vi "FTW-Project-ConditionalDisableSymbols-Set.vi"(0 "Project Ref (blank for Active Project)":refnum<vi>, 5 "Target (Root or My Computer)":string(combo)="Root", 7 "Conditional Disable Symbol":string, 9 "Value":string, 11 "error in":errorcluster) -> (4 "Project out":refnum<vi>, 6 "Conditional Disable Symbols out":variant, 15 "error out":errorcluster)   [LabVIEW 2012]
doc: "This VI will add to or modify existing Conditional Disable Symbols. It will not remove existing Conditional Disable Symbols."
panel:
  # "Inputs"
  # "Outputs"
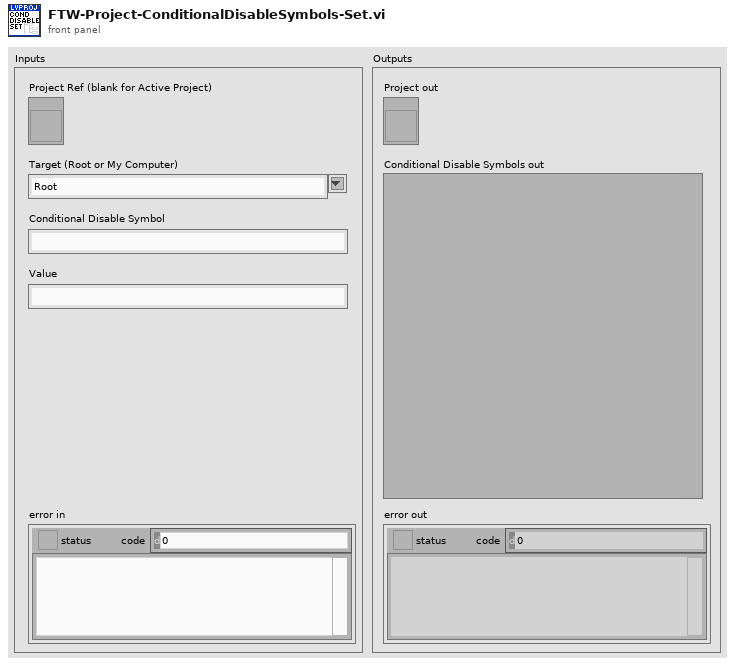
[diagram p1: front panel]
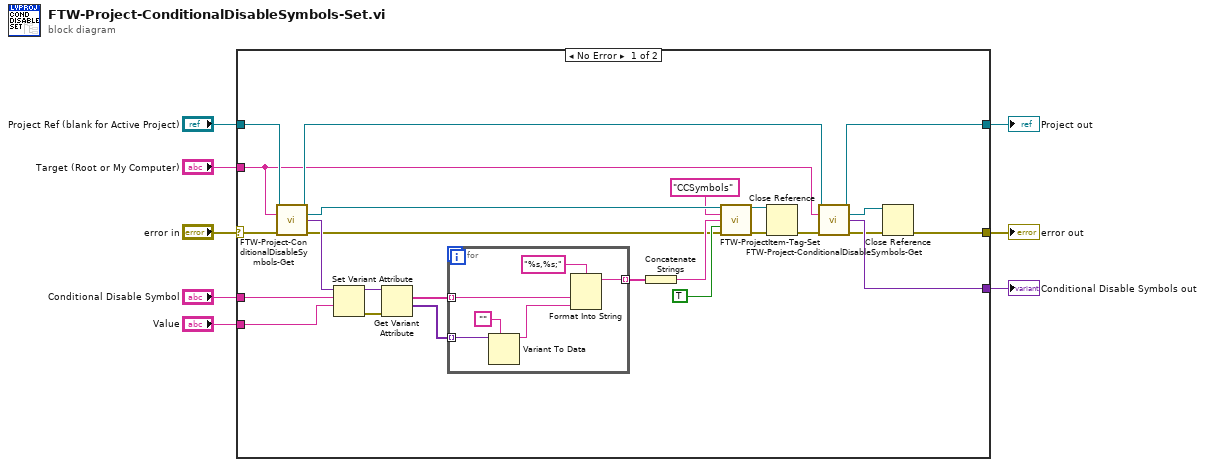
[diagram p0: block diagram]
diagram:
  n1 = case shown="No Error" "error in" {
    selector: "error in" -> [w32 w41]
    tunnel: [w19 w41] -> w8
    tunnel: "Target (Root or My Computer)" -> [w23 _]
    tunnel: "Project Ref (blank for Active Project)" -> [w33 w40]
    tunnel: [w25 w40] -> w4
    tunnel: [w22 _] -> w3
    tunnel: "Conditional Disable Symbol" -> [w18 _]
    tunnel: "Value" -> [w17 _]
    frame No Error {
      n2 = call "FTW-Project-ConditionalDisableSymbols-Get.vi"("Project Ref (blank for Active Project)"=w33, "Target (Root or My Computer)"=w23, "error in"=w32) -> ("Project out"=w26:refnum<vi>, "TargetItem out"=w16:refnum<vi>, "Conditional Disable Symbols"=w31:variant, "error out"=w12:errorcluster)  [unwired: 9 in]
      n3 = Set Variant Attribute(Variant=w31, name=w18, value=w17) -> (Variant out=w30:variant, error out=w9:errorcluster)  [unwired: 1 in, 1 out]
      n4 = Get Variant Attribute(Variant=w30, error in=w9) -> (names=w29:string[], values=w28:variant[])  [unwired: 2 in, 2 out]
      n5 = for {
        tunnel: w29 -> [w35] mode=indexing
        tunnel: w28 -> [w39] mode=indexing
        tunnel: [w34] -> w27 mode=indexing
        n6 = Variant To Data(type="", Variant=w39) -> (data=w36:string)  [unwired: 1 in, 1 out]
        n7 = Format Into String(format string="%s,%s;", w35, w36) -> (resulting string=w34:string)  [unwired: 2 in, 1 out]
      }
      n8 = Concatenate Strings(w27) -> (w14:string)
      n9 = call "FTW-ProjectItem-Tag-Set.vi"("ProjectItem"=w16, "Tag Name"="CCSymbols", "Tag Value"=w14, "Persistent?"=TRUE ("Is Persistent"), "error in"=w12) -> ("ProjectItem out"=w10:refnum<vi>, "error out"=w11:errorcluster)  [unwired: 9 in]
      n10 = Close Reference(reference=w10, error in (no error)=w11) -> (error out=w24:errorcluster)
      n11 = call "FTW-Project-ConditionalDisableSymbols-Get.vi"("Project Ref (blank for Active Project)"=w26, "Target (Root or My Computer)"=w23, "error in"=w24) -> ("Project out"=w25:refnum<vi>, "TargetItem out"=w21:refnum<vi>, "Conditional Disable Symbols"=w22:variant, "error out"=w20:errorcluster)  [unwired: 9 in]
      n12 = Close Reference(reference=w21, error in (no error)=w20) -> (error out=w19:errorcluster)
    }
    frame Error {
    }
  }
  "error out" <- w8
  "Project out" <- w4
  "Conditional Disable Symbols out" <- w3
